vi "Shift_001.vi"() -> ()   [LabVIEW 2019]
panel:
  out "Numeric":dbl
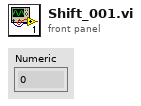
[diagram p1: front panel]
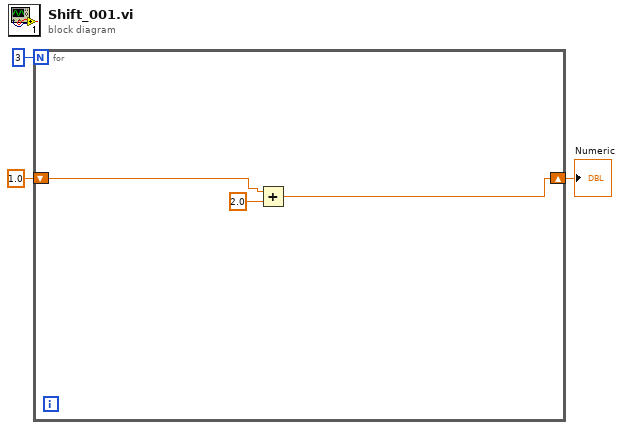
[diagram p0: block diagram]
diagram:
  n1 = for {
    N: 3 -> [_]
    shift-right: [w5] -> w1
    shift-left: 1.0 -> [w6]
    n2 = Add(x=w6, y=2.0) -> (x+y=w5:dbl)
  }
  "Numeric" <- w1
